vi "_PutData.vi"(8 "Error In":errorcluster, 9 "Byte Array":u8[](array[numeric]), 10 "Index Or Position":u32, 11 "ByteBuffer In":refnum<class "ByteBuffer.lvclass">) -> (0 "Error Out":errorcluster, 3 "ByteBuffer Out":refnum<class "ByteBuffer.lvclass">)   [LabVIEW 2015, in "ByteBuffer.lvclass"]
uses:
  ByteBuffer.lvclass
  ByteBuffer.lvclass/ByteBuffer.ctl
  properties/position/Set Position.vi
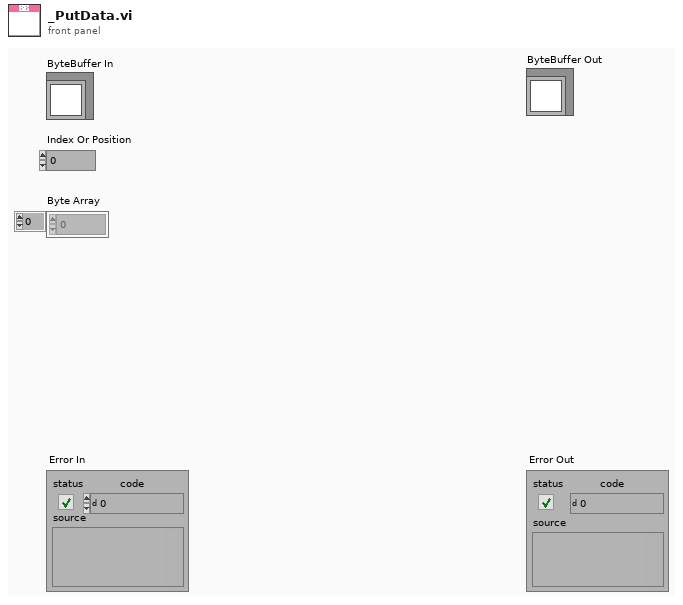
[diagram p1: front panel]
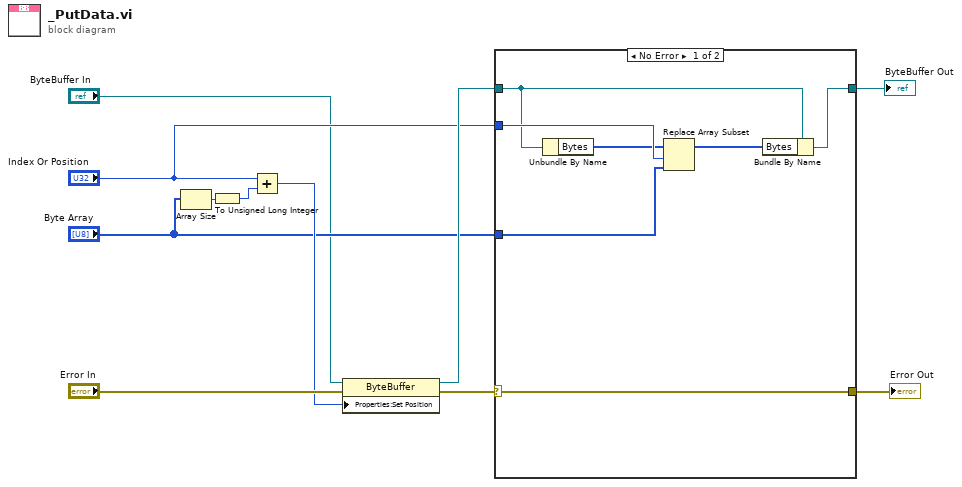
[diagram p0: block diagram]
diagram:
  n1 = Array Size(array="Byte Array") -> (size(s)=w8:i32)
  n2 = To Unsigned Long Integer(number=w8) -> (unsigned 32bit integer=w7:u32)
  n3 = Add(x="Index Or Position", y=w7) -> (x+y=w4:u32)
  n4 = property class="ByteBuffer"(reference="ByteBuffer In", error in="Error In", "Properties:Set Position"=w4) -> (reference out=w6:refnum<class "ByteBuffer.lvclass">, error out=w5:errorcluster)
  n5 = case shown="No Error" w5 {
    selector: w5 -> [w18 w20]
    tunnel: w6 -> [w13 w19]
    tunnel: [w18 w20] -> w10
    tunnel: [w16 w19] -> w9
    tunnel: "Index Or Position" -> [w15 _]
    tunnel: "Byte Array" -> [w14 _]
    frame No Error {
      n6 = Unbundle By Name(w13) -> ("Bytes"=w12:u8[])
      n7 = Replace Array Subset(array=w12, new element=w14, index=w15) -> (w17:u8[])
      n8 = Bundle By Name(cluster=w13, "Bytes"=w17) -> (w16:refnum<class "ByteBuffer.lvclass">)
    }
    frame Error {
    }
  }
  "Error Out" <- w10
  "ByteBuffer Out" <- w9
